vi "Convert Volts to dBV.vi"(4 "Volts":dbl format="%.2f") -> (1 "dBV":dbl format="%.2f")   [LabVIEW 2011]
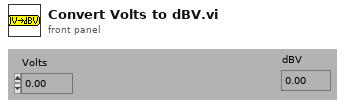
[diagram p1: front panel]
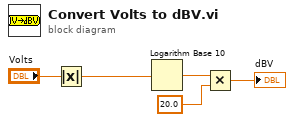
[diagram p0: block diagram]
diagram:
  n1 = Absolute Value(x="Volts") -> (abs(x)=w1:dbl)
  n2 = Logarithm Base 10(1:w1) -> (0:w5:dbl)
  n3 = Multiply(x=w5, y=20.0) -> (x*y=→"dBV":dbl)
